vi "Logger_Init.vi"(7 "CAlexVersion":T1=enum."Mobile", 8 "error in (no error)":errorcluster, 9 "SyncOut":refnum<k21>, 10 "SyncIn":refnum<k21>="SyncIn_Vicon") -> (0 "error out":errorcluster, 3 "Logger Loop Cluster":T2={"Data Logger out"=refnum, "CAlexVersion"=enum."Mobile", "SyncIn"="", "SyncOut"=""})   [LabVIEW 2016]
uses:
  Logger Cluster.ctl
  Classes/DataLogger/Data Logger.lvclass
  Classes/CAlex2/TypeDef/CAlexVersion.ctl
  <vilib>/DAQmx/write.llb/DAQmx Write (Digital Bool 1Line 1Point).vi
  <vilib>/DAQmx/miscellaneous.llb/DAQmx Fill In Error Info.vi
  Classes/CAlex2/CAlex2.lvclass
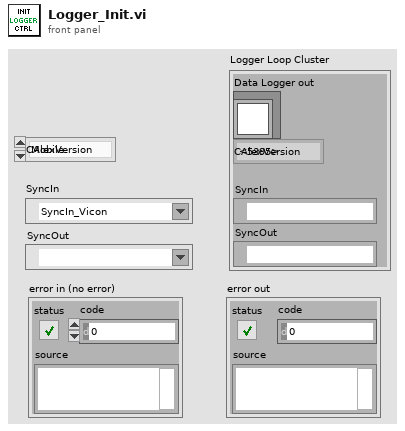
[diagram p1: front panel]
types:
  T1 = typedef "CAlex2.lvclass/CAlexVersion.ctl" = enum16{"Bilateral_Squat", "Squat", "Treadmill", "Mobile"}
  T2 = typedef "Logger Cluster.ctl" = cluster{"Data Logger out":refnum<class "Data Logger.lvclass">, "CAlexVersion":T1, "SyncIn":refnum<k21>, "SyncOut":refnum<k21>}
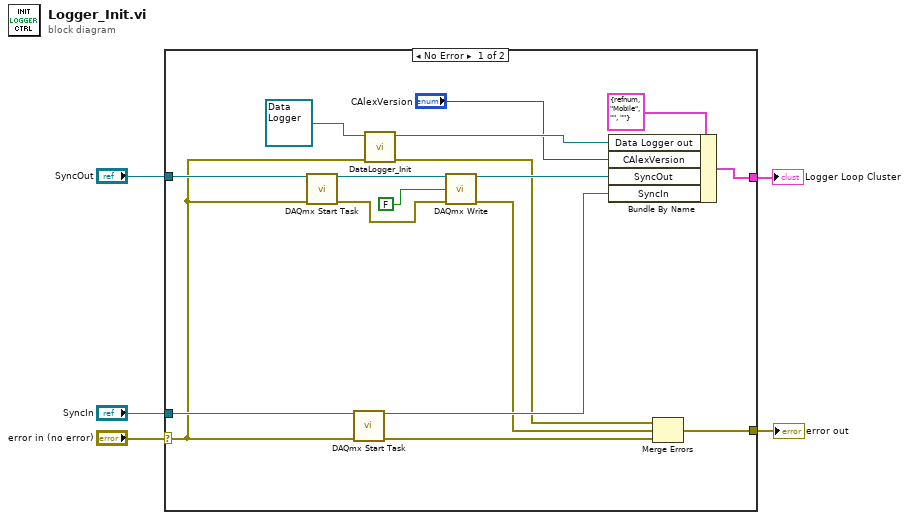
[diagram p0: block diagram]
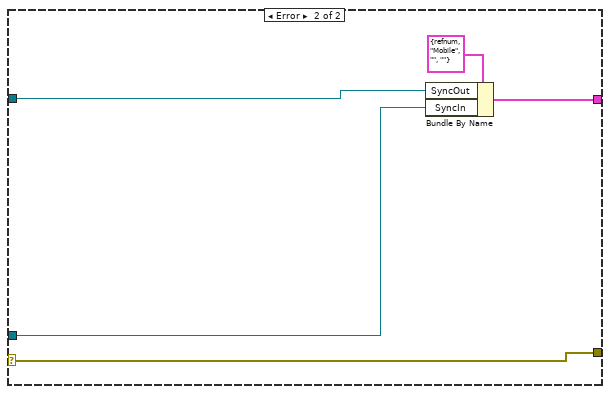
[diagram p2: hidden frame]
diagram:
  n1 = case shown="No Error" "error in (no error)" {
    selector: "error in (no error)" -> [w8 w27]
    tunnel: [w21 w27] -> w5
    tunnel: "SyncIn" -> [w19 w25]
    tunnel: "SyncOut" -> [w16 w24]
    tunnel: [w11 w23] -> w2
    frame No Error {
      n2 = call <vilib>:"DAQmx Start Task.vi"("task/channels in"=w16, "error in"=w8) -> ("task out"=w18:refnum<k21>, "error out"=w20:errorcluster)  [unwired: 12 in]
      n3 = call <vilib>:"DAQmx Start Task.vi"("task/channels in"=w19, "error in"=w8) -> ("task out"=w13:refnum<k21>, "error out"=w22:errorcluster)  [unwired: 12 in]
      n4 = call "DataLogger_Init.vi"("error in (no error)"=w8, "Data Logger in"=refnum<class "Data Logger.lvclass"> refnum ("Data Logger.lvclass")) -> ("error out"=w9:errorcluster, "Data Logger out"=w7:refnum<class "Data Logger.lvclass">)  [unwired: 8 in]
      n5 = call-poly <vilib>:"DAQmx Write.vi"("task/channels in"=w18, "data"=FALSE, "error in"=w20) -> ("task out"=w12:refnum<k21>, "error out"=w10:errorcluster)  [unwired: 10 in, 1 out]
      n6 = Bundle By Name(cluster=T2 {"Data Logger out"=refnum, "CAlexVersion"=enum."Mobile", "SyncIn"="", "SyncOut"=""} ("Logger Loop Cluster"), "Data Logger out"=w7, "CAlexVersion"="CAlexVersion", "SyncOut"=w12, "SyncIn"=w13) -> (w11:T2)
      n7 = Merge Errors(w9, w10, w22) -> (w21:errorcluster)
    }
    frame Error {
      n8 = Bundle By Name(cluster=T2 {"Data Logger out"=refnum, "CAlexVersion"=enum."Mobile", "SyncIn"="", "SyncOut"=""} ("Logger Loop Cluster"), "SyncOut"=w24, "SyncIn"=w25) -> (w23:T2)
    }
  }
  "error out" <- w5
  "Logger Loop Cluster" <- w2
